vi "parse standard name.vi"(7 "standard name":string, 8 "error in":errorcluster, 9 "zero index bit":bool, 10 "zero index element":bool, 11 "Modbus Module Channel in":refnum<class "Modbus Module Channel.lvclass">) -> (0 "error out":errorcluster, 3 "Modbus Module Channel out":refnum<class "Modbus Module Channel.lvclass">)   [LabVIEW 2015, in "Modbus Module Channel.lvclass"]
uses:
  Modbus Module Channel.lvclass
  data bank type.ctl
  Modbus Module Channel.lvclass/Modbus Module Channel.ctl
  Write modbus type.vi
  Write starting address.vi
  Write subindex (bool).vi
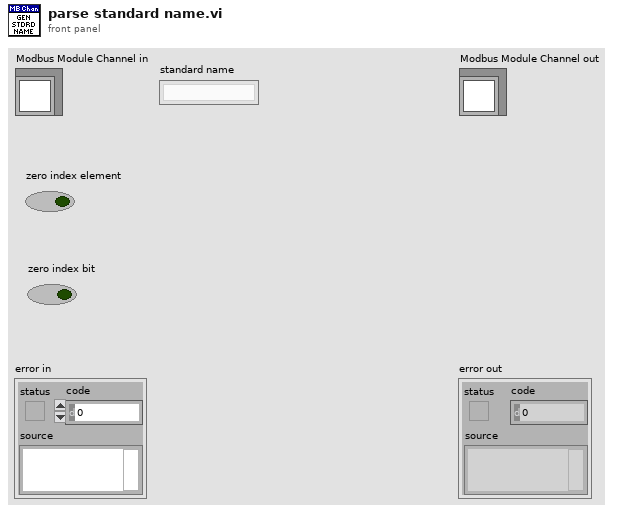
[diagram p1: front panel]
types:
  T1 = typedef "Modbus Module Channel.lvclass/data bank type.ctl" = enum16{"Coils", "Discrete Inputs", "Input Registers", "Holding Registers"}
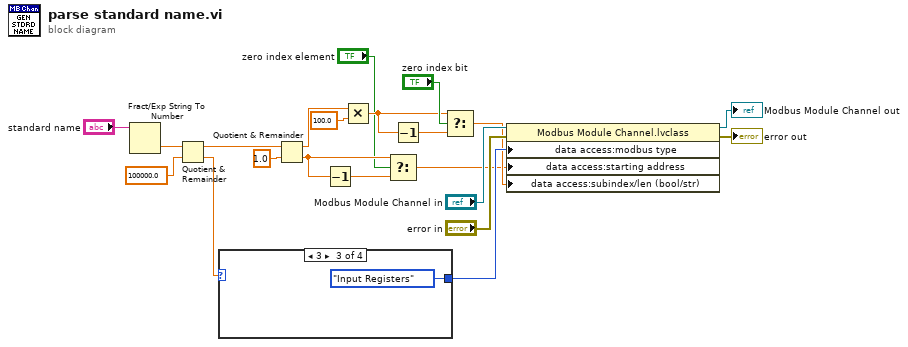
[diagram p0: block diagram]
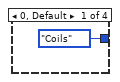
[diagram p2: hidden frame]
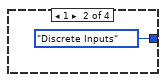
[diagram p3: hidden frame]
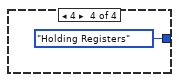
[diagram p4: hidden frame]
diagram:
  n1 = Fract/Exp String To Number(string="standard name") -> (number=w20:dbl)  [unwired: 3 in, 1 out]
  n2 = Quotient & Remainder(x=w20, y=100000.0) -> (x-y*floor(x/y)=w17:dbl, floor(x/y)=w18:dbl)
  n3 = case shown="3" w18 {
    tunnel: [data_bank_type."Coils" ("modbus type") data_bank_type."Discrete Inputs" ("modbus type") data_bank_type."Input Registers" ("modbus type") data_bank_type."Holding Registers" ("modbus type")] -> w3
    frame 0, Default {
    }
    frame 1 {
    }
    frame 3 {
    }
    frame 4 {
    }
  }
  n4 = Quotient & Remainder(x=w17, y=1.0) -> (x-y*floor(x/y)=w15:dbl, floor(x/y)=w9:dbl)
  n5 = Decrement(x=w9) -> (x-1=w10:dbl)
  n6 = Multiply(x=w15, y=100.0) -> (x*y=w12:dbl)
  n7 = Select(t=w9, s="zero index element", f=w10) -> (s? t:f=w1:dbl)
  n8 = Decrement(x=w12) -> (x-1=w11:dbl)
  n9 = Select(t=w12, s="zero index bit", f=w11) -> (s? t:f=w2:dbl)
  n10 = property class="Modbus Module Channel.lvclass"(reference="Modbus Module Channel in", error in="error in", "data access:modbus type"=w3, "data access:starting address"=w1, "data access:subindex/len (bool/str)"=w2) -> (reference out=→"Modbus Module Channel out":refnum<class "Modbus Module Channel.lvclass">, error out=→"error out":errorcluster)
